vi "Close.vi"(8 "error in (no error)":errorcluster, 11 "Wifi in":refnum<class "Wifi.lvclass">) -> (0 "error out":errorcluster, 3 "Wifi out":refnum<class "Wifi.lvclass">)   [LabVIEW 2021, in "Wifi.lvclass"]
uses:
  Wifi.lvclass
  Wifi.lvclass/Wifi.ctl
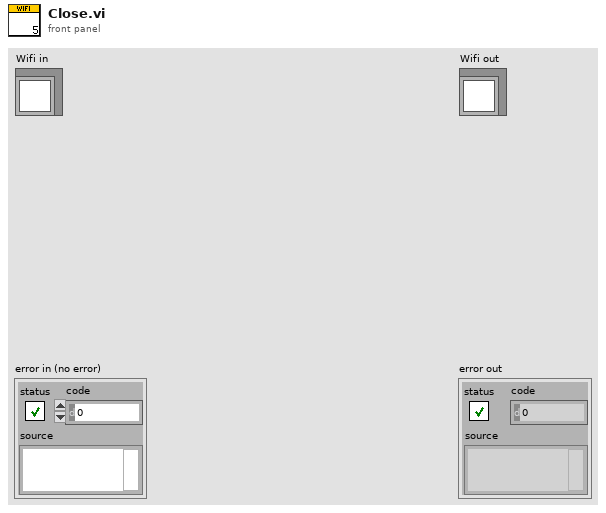
[diagram p1: front panel]
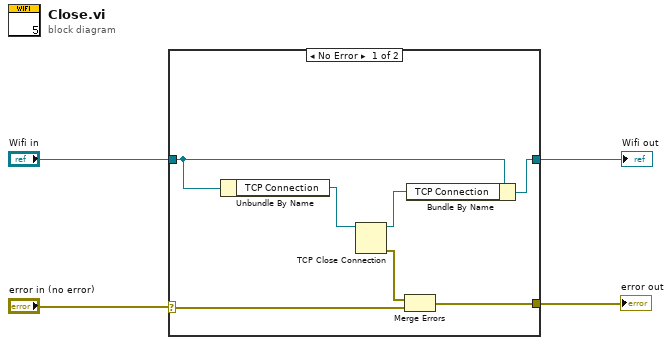
[diagram p0: block diagram]
diagram:
  n1 = case shown="No Error" "error in (no error)" {
    selector: "error in (no error)" -> [w11 w12]
    tunnel: [w9 w12] -> w3
    tunnel: "Wifi in" -> [w7 w13]
    tunnel: [w5 w13] -> w1
    frame No Error {
      n2 = Unbundle By Name(w7) -> ("TCP Connection"=w8:refnum<k5>)
      n3 = TCP Close Connection(connection ID=w8) -> (connection ID out=w6:refnum<k5>, error out=w10:errorcluster)  [unwired: 1 in, 1 out]
      n4 = Merge Errors(w10, w11) -> (w9:errorcluster)
      n5 = Bundle By Name(cluster=w7, "TCP Connection"=w6) -> (w5:refnum<class "Wifi.lvclass">)
    }
    frame Error {
    }
  }
  "error out" <- w3
  "Wifi out" <- w1
